vi "SaveCamConfig-v5.vi"(0 "file path in":path, 2 "CamConfigArray":T2(array[cluster]) {"CorrectConfig Cluster"."Acquisition Parameters"."White level" scale=0.3..1.26 scale format="%#_2f"; "CorrectConfig Cluster"."Acquisition Parameters"."Saturation" scale=0.5..1.5 scale format="%#_3f"; "CorrectConfig Cluster"."Acquisition Parameters"."Contrast" scale=0.4..1.5 scale format="%#_3f"; "CorrectConfig Cluster"."Acquisition Parameters"."Brightness" scale=-50.0..50.0 scale format="%#_2f"; "CorrectConfig Cluster"."Correction Parameters"."Movement Type" items=["Step", "Proportionnal"]; "CorrectConfig Cluster"."Target"."X Target" format="%#_5g"; "CorrectConfig Cluster"."Target"."Y Target" format="%#_5g"; "CorrectConfig Cluster"."Detection Parameters"."Max Intensity%" max=100 step=1}) -> (8 "parse errors":string)   [LabVIEW 2013]
uses:
  <vilib>/userdefined/High Color/IMAQdx.ctl
panel:
  out "DeviceList":T3(array[cluster]) {"Acquisition Parameters"."White level" scale=0.3..1.26 scale format="%#_2f"; "Acquisition Parameters"."Saturation" scale=0.5..1.5 scale format="%#_3f"; "Acquisition Parameters"."Contrast" scale=0.4..1.5 scale format="%#_3f"; "Acquisition Parameters"."Brightness" scale=-50.0..50.0 scale format="%#_2f"; "Correction Parameters"."Movement Type" items=["Step", "Proportionnal"]; "Target"."X Target" format="%#_5g"; "Target"."Y Target" format="%#_5g"; "Detection Parameters"."Max Intensity%" max=100 step=1}
  out "Numeric":i32
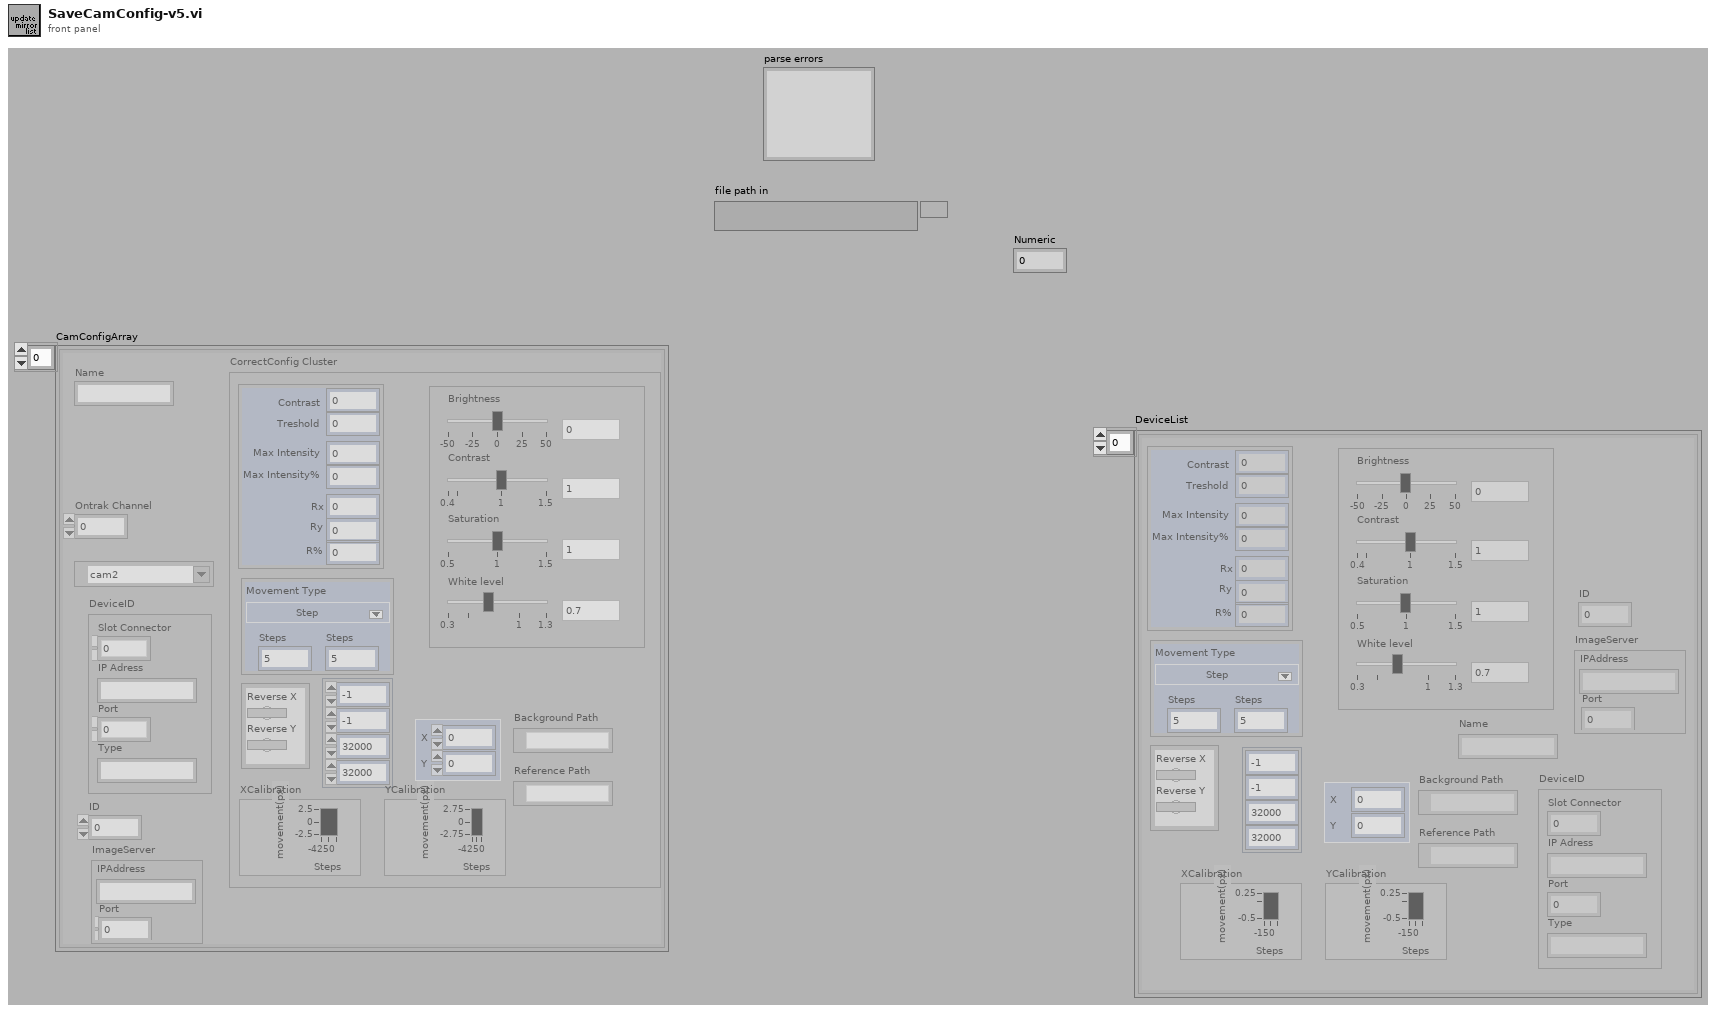
[diagram p1: front panel]
types:
  T1 = typedef "IMAQdx.ctl" = refnum<k21>
  T2 = cluster{"ID":dbl, "Name":string, "DeviceID":cluster{"Slot Connector":i32, "IP Adress":string, "Port":i32, "Type":string}, "CorrectConfig Cluster":cluster{"Detection Parameters":cluster{"Contrast":i32, "Treshold":u8, "Max Intensity":i32, "Max Intensity%":u8, "Rx":i32, "Ry":i32, "R%":sgl}, "Reverse":cluster{"Reverse X":bool, "Reverse Y":bool}, "Target":cluster{"X Target":sgl, "Y Target":sgl}, "Region of Interest":i32[], "Correction Parameters":cluster{"X":sgl, "Y":sgl, "Movement Type":u16}, "Acquisition Parameters":cluster{"Brightness":dbl, "Contrast":dbl, "Saturation":dbl, "White level":dbl}, "Background Path":path, "Reference Path":path, "XCalibration":cluster{dbl, dbl}[], "YCalibration":cluster{dbl, dbl}[]}, "Ontrak Channel":i16, "IMAQdx Session":T1, "ImageServer":cluster{"IPAddress":string, "Port":i32}}[]
  T3 = cluster{"ID":dbl, "Name":string, "DeviceID":cluster{"Slot Connector":i32, "IP Adress":string, "Port":i32, "Type":string}, "Detection Parameters":cluster{"Contrast":i32, "Treshold":u8, "Max Intensity":i32, "Max Intensity%":u8, "Rx":i32, "Ry":i32, "R%":sgl}, "Reverse":cluster{"Reverse X":bool, "Reverse Y":bool}, "Target":cluster{"X Target":sgl, "Y Target":sgl}, "Region of Interest":i32[], "Correction Parameters":cluster{"X":sgl, "Y":sgl, "Movement Type":u16}, "Acquisition Parameters":cluster{"Brightness":dbl, "Contrast":dbl, "Saturation":dbl, "White level":dbl}, "Background Path":path, "Reference Path":path, "XCalibration":cluster{dbl, dbl}[], "YCalibration":cluster{dbl, dbl}[], "ImageServer":cluster{"IPAddress":string, "Port":i32}}[]
  T4 = cluster{"Slot Connector":i32, "IP Adress":string, "Port":i32, "Type":string}
  T5 = cluster{"Detection Parameters":cluster{"Contrast":i32, "Treshold":u8, "Max Intensity":i32, "Max Intensity%":u8, "Rx":i32, "Ry":i32, "R%":sgl}, "Reverse":cluster{"Reverse X":bool, "Reverse Y":bool}, "Target":cluster{"X Target":sgl, "Y Target":sgl}, "Region of Interest":i32[], "Correction Parameters":cluster{"X":sgl, "Y":sgl, "Movement Type":u16}, "Acquisition Parameters":cluster{"Brightness":dbl, "Contrast":dbl, "Saturation":dbl, "White level":dbl}, "Background Path":path, "Reference Path":path, "XCalibration":cluster{dbl, dbl}[], "YCalibration":cluster{dbl, dbl}[]}
  T6 = cluster{"Contrast":i32, "Treshold":u8, "Max Intensity":i32, "Max Intensity%":u8, "Rx":i32, "Ry":i32, "R%":sgl}
  T7 = cluster{"Brightness":dbl, "Contrast":dbl, "Saturation":dbl, "White level":dbl}
  T8 = cluster{"ID":dbl, "Name":string, "DeviceID":cluster{"Slot Connector":i32, "IP Adress":string, "Port":i32, "Type":string}, "Detection Parameters":cluster{"Contrast":i32, "Treshold":u8, "Max Intensity":i32, "Max Intensity%":u8, "Rx":i32, "Ry":i32, "R%":sgl}, "Reverse":cluster{"Reverse X":bool, "Reverse Y":bool}, "Target":cluster{"X Target":sgl, "Y Target":sgl}, "Region of Interest":i32[], "Correction Parameters":cluster{"X":sgl, "Y":sgl, "Movement Type":u16}, "Acquisition Parameters":cluster{"Brightness":dbl, "Contrast":dbl, "Saturation":dbl, "White level":dbl}, "Background Path":path, "Reference Path":path, "XCalibration":cluster{dbl, dbl}[], "YCalibration":cluster{dbl, dbl}[], "ImageServer":cluster{"IPAddress":string, "Port":i32}}
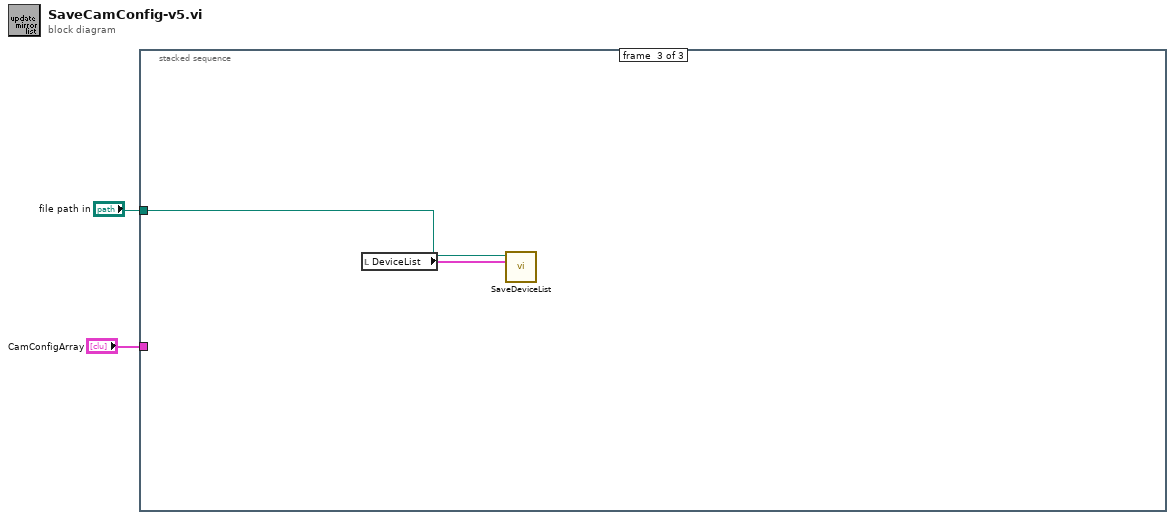
[diagram p0: block diagram]
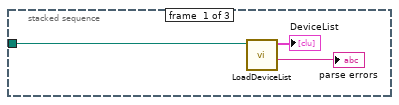
[diagram p2: hidden frame]
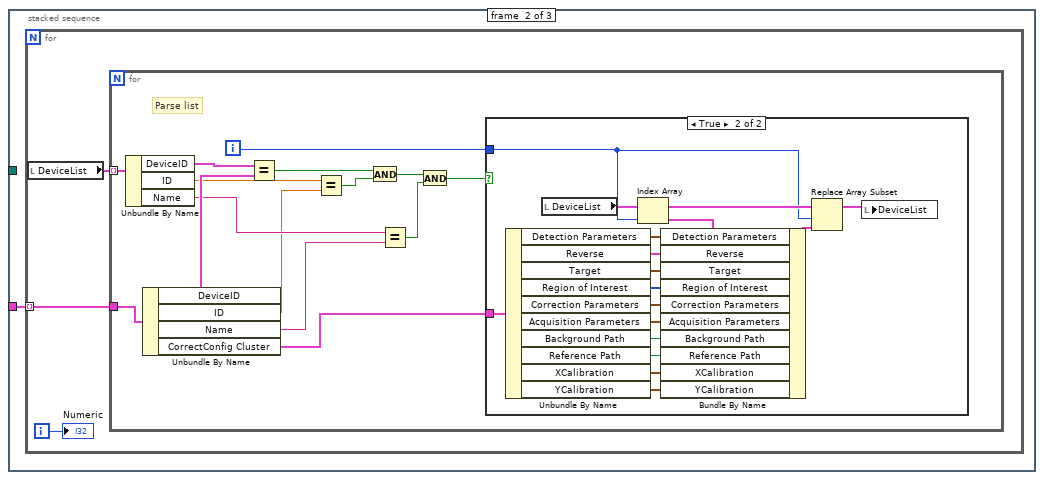
[diagram p3: hidden frame]
diagram:
  n1 = stacked-sequence {
    tunnel: "file path in" -> [w5 _ w41]
    tunnel: "CamConfigArray" -> [_ w6 _]
    frame #0 {
      n2 = call "LoadDeviceList.vi"("path to XML document"=w5) -> ("parse errors"=→"parse errors":string, "DeviceList"=→"DeviceList":T3)  [unwired: 8 in, 1 out]
    }
    frame #1 {
      n3 = for {
        tunnel: w6 -> [w8] mode=indexing
        i -> [w9]
        n4 = local read "DeviceList"() -> (w7:T3)
        n5 = for {
          tunnel: w8 -> [w23]
          tunnel: w7 -> [w22] mode=indexing
          i -> [w20]
          # "Parse list"
          n6 = Unbundle By Name(w22) -> ("DeviceID"=w21:T4, "ID"=w17:dbl, "Name"=w16:string)
          n7 = Unbundle By Name(w23) -> ("DeviceID"=w24:T4, "ID"=w15:dbl, "Name"=w14:string, "CorrectConfig Cluster"=w19:T5)
          n8 = Equal?(x=w21, y=w24) -> (x = y?=w18:bool)
          n9 = Equal?(x=w17, y=w15) -> (x = y?=w13:bool)
          n10 = And(x=w18, y=w13) -> (x .and. y?=w10:bool)
          n11 = Equal?(x=w16, y=w14) -> (x = y?=w12:bool)
          n12 = And(x=w10, y=w12) -> (x .and. y?=w11:bool)
          n13 = case shown="True" w11 {
            tunnel: w19 -> [_ w37]
            tunnel: w20 -> [_ w38]
            frame False {
            }
            frame True {
              n14 = Unbundle By Name(w37) -> ("Detection Parameters"=w34:T6, "Reverse"=w33:cluster{"Reverse X":bool, "Reverse Y":bool}, "Target"=w32:cluster{"X Target":sgl, "Y Target":sgl}, "Region of Interest"=w31:i32[], "Correction Parameters"=w30:cluster{"X":sgl, "Y":sgl, "Movement Type":u16}, "Acquisition Parameters"=w29:T7, "Background Path"=w28:path, "Reference Path"=w27:path, "XCalibration"=w26:cluster{dbl, dbl}[], "YCalibration"=w25:cluster{dbl, dbl}[])
              n15 = local read "DeviceList"() -> (w40:T3)
              n16 = Index Array(array=w40, index=w38) -> (element=w36:T8)
              n17 = Bundle By Name(cluster=w36, "Detection Parameters"=w34, "Reverse"=w33, "Target"=w32, "Region of Interest"=w31, "Correction Parameters"=w30, "Acquisition Parameters"=w29, "Background Path"=w28, "Reference Path"=w27, "XCalibration"=w26, "YCalibration"=w25) -> (w35:T8)
              n18 = Replace Array Subset(array=w40, new element=w35, index=w38) -> (w39:T3)
              n19 = local write "DeviceList"(w39) -> ()
            }
          }
        }
        "Numeric" <- w9
      }
    }
    frame #2 {
      n20 = local read "DeviceList"() -> (w42:T3)
      n21 = call "SaveDeviceList.vi"("DeviceList"=w42, "path to XML document"=w41) -> ()  [unwired: 8 in, 2 out]
    }
  }
